vi "VCS Get Encoder Parameter.vi"(8 "error in (no error)":errorcluster, 11 "axis in":cluster{"keyHandle":u32, "nodeId":u16}={"keyHandle"=0, "nodeId"=1}) -> (0 "error out":errorcluster, 2 "encoder parameter":cluster{"sensorType":u16, "encoder counts":u16}={"sensorType"=1, "encoder counts"=500} {"sensorType" items=["Incremental Encoder (3 Channel)"=1, "Incremental Encoder (2 Channel)"=2, "Halls Sensors"=3]}, 3 "axis out":cluster{"keyHandle":u32, "nodeId":u16}={"keyHandle"=0, "nodeId"=1})   [LabVIEW 2010]
doc: "<B>VCS Get Encoder Parameter</B> reads all encoder parameters."
uses:
  Resources/EposCmd.dll
  Resources/EposCmd64.dll
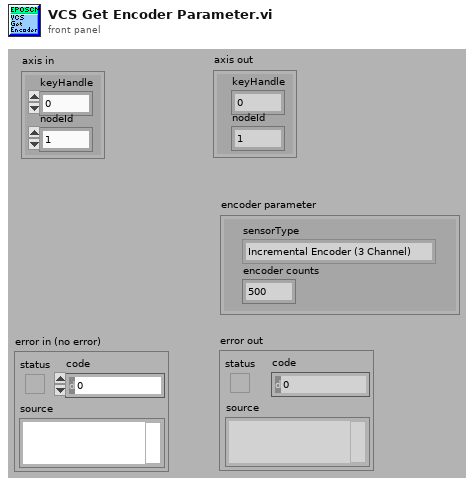
[diagram p1: front panel]
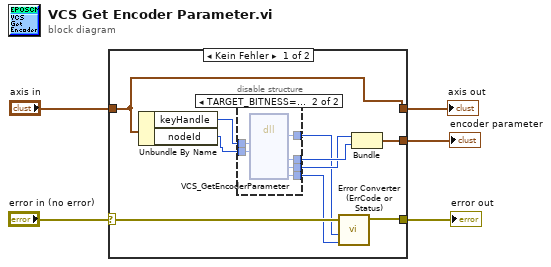
[diagram p0: block diagram]
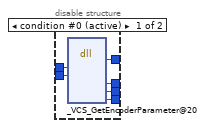
[diagram p2: hidden frame]
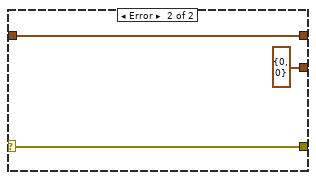
[diagram p3: hidden frame]
diagram:
  n1 = case shown="Kein Fehler" "error in (no error)" {
    selector: "error in (no error)" -> [w15 w30]
    tunnel: [w14 w30] -> w4
    tunnel: "axis in" -> [w7 w29]
    tunnel: [w8 cluster{"pSensorType":u16, "pCounts":u16} {"pSensorType"=0, "pCounts"=0}] -> w2
    tunnel: [w7 w29] -> w1
    frame No Error {
      n2 = Unbundle By Name(w7) -> ("keyHandle"=w12:u32, "nodeId"=w11:u16)
      n3 = disable-structure shown="TARGET_BITNESS==64" {
        disable-tunnel: [w21 w27] -> w13
        disable-tunnel: w12 -> [w20 w26]
        disable-tunnel: w11 -> [w19 w25]
        disable-tunnel: [w18 w24] -> w10
        disable-tunnel: [w17 w23] -> w9
        disable-tunnel: [w16 w22] -> w6
        frame condition #0 (active) {
          n4 = dll-call lib="C:/Sources/LabView/maxon EPOS/Resources/EposCmd.*" fn="_VCS_GetEncoderParameter@20"("KeyHandle"=w20, "NodeId"=w19) -> (w16:i32, "pCounts"=w18:u16, "pSensorType"=w17:u16, "pErrorCode"=w21:u32)  [unwired: 8 in, 2 out]
        }
        frame condition #1 {
          n5 = dll-call lib="C:/setup/Resources/EposCmd64.*" fn="VCS_GetEncoderParameter" ("EposCmd.dll:_VCS_GetEncoderParameter@20")("KeyHandle"=w26, "NodeId"=w25) -> ("Rückgabetyp"=w22:i32, "pCounts"=w24:u16, "pSensorType"=w23:u16, "pErrorCode"=w27:u32)  [unwired: 8 in, 2 out]
        }
      }
      n6 = call "Error Converter (ErrCode or Status).vi"("error code"=w13, "return type"=w6, "error in (no error)"=w15) -> ("error out"=w14:errorcluster)  [unwired: 7 in]
      n7 = Bundle("pSensorType"=w9, "pCounts"=w10) -> (w8:cluster{"pSensorType":u16, "pCounts":u16})  [unwired: 1 in]
    }
    frame Error {
    }
  }
  "error out" <- w4
  "encoder parameter" <- w2
  "axis out" <- w1
